vi "enumerateStaticDependencies.vi"(8 "error in (no error)":errorcluster, 11 "SMO.Activity":refnum<class "SMO.Activity.lvclass">) -> (0 "error out":errorcluster, 2 "Static Dependencies":refnum<class "Dependency.lvclass">[](array[class]), 3 "SMO.Activity out":refnum<class "SMO.Activity.lvclass">)   [LabVIEW 2015, in "SMO.Activity.lvclass"]
doc: "JKI State Machine Objects (SMO) 1.1.8.32\nJKI - JKI\nCopyright (c) 2016, JKI"
uses:
  SMO.Activity.lvclass
  <vilib>/JKI/JKI SMO/Dependency/Dependency.lvclass
  <vilib>/JKI/JKI SMO/SMO/SMO.lvclass
panel:
  # "For instructions on how to use the JKI State Machine Objects, examples and video tutorials, visit:\nhttp://jki.net/state-machine-objects/\n\nJKI State Machine Objects™\nhttp://jki.net/state-machine-objects/\nCopyright (C) 2005-2015, JKI <info@jki.net>\nALL RIGHTS RESERVED"
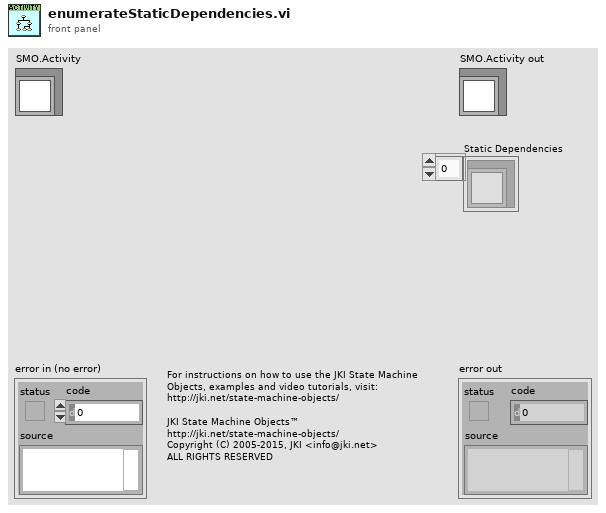
[diagram p1: front panel]
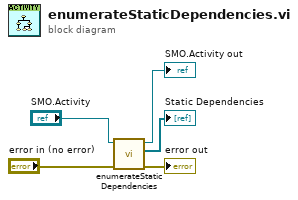
[diagram p0: block diagram]
diagram:
  n1 = call-parent "enumerateStaticDependencies.vi"("error in (no error)"="error in (no error)", "SMO"="SMO.Activity") -> ("error out"=→"error out":errorcluster, "Static Dependencies"=→"Static Dependencies":refnum<class "Dependency.lvclass">[], "SMO out"=→"SMO.Activity out":refnum<class "SMO.Activity.lvclass">)  [unwired: 7 in]
